vi "Set Defaults.vi"(11 "NewEntityTemplate in":refnum<class "LiveDemo.lvclass">) -> (3 "NewEntityTemplate out":refnum<class "LiveDemo.lvclass">)   [LabVIEW 2020, in "tests.lvlib" / "LiveDemo.lvclass"]
uses:
  LiveDemo.lvclass
  LiveDemo.lvclass/LiveDemo.ctl
  <vilib>/IlluminatedG/IG Conditum Base/Conditum/Columns/Integer/Integer.lvclass
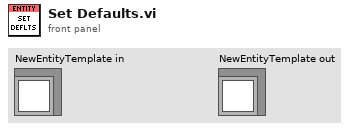
[diagram p1: front panel]
types:
  T1 = typedef "tests.lvlib/LiveDemo.lvclass/Columns.ctl" = cluster{"<Placeholder>":refnum<class "Integer.lvclass">}
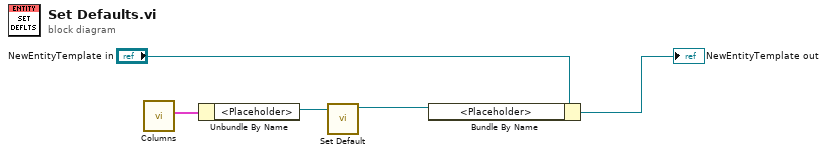
[diagram p0: block diagram]
diagram:
  n1 = call "Columns.vi"() -> ("Columns"=w2:T1)  [unwired: 11 in]
  n2 = Unbundle By Name(w2) -> ("<Placeholder>"=w3:refnum<class "Integer.lvclass">)
  n3 = call-dynamic "Set Default.vi"("Integer in"=w3) -> ("Integer out"=w1:refnum<class "Integer.lvclass">)  [unwired: 10 in]
  n4 = Bundle By Name(cluster="NewEntityTemplate in", "<Placeholder>"=w1) -> (→"NewEntityTemplate out":refnum<class "LiveDemo.lvclass">)
